vi "Close.vi"(8 "error in (no error)":errorcluster, 11 "Mercury Reference":T1) -> (0 "error out":errorcluster)   [LabVIEW 2019, in "Mercury iXX.lvlib"]
doc: "Close the Mercury reference to the instrument. This will close the physcial communication layer.\nPlease use this only once at the end of your application."
uses:
  Mercury iXX.lvlib
  Controls/Mercury Reference.ctl
  Controls/Comms Transport Layer.ctl
  Private/Controls/Query Dynamic Reference.ctl
  Private/Controls/Lookup Reference FGV Enum.ctl
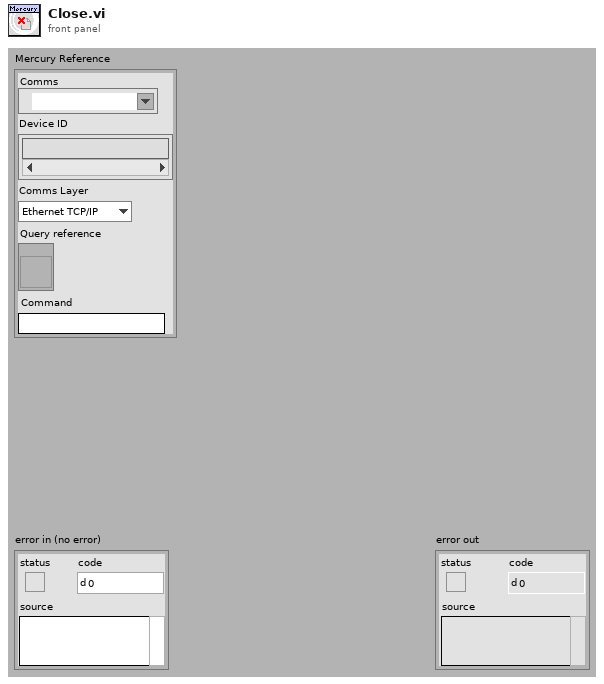
[diagram p1: front panel]
types:
  T1 = typedef "Mercury iXX.lvlib/Mercury Reference.ctl" = cluster{"Comms":refnum<visa-resource-name>, "Device ID":string[], "Comms Layer":T2, "Command":string, "Query reference":T3}
  T2 = typedef "Mercury iXX.lvlib/Comms Transport Layer.ctl" = enum16{"Ethernet TCP/IP", "USB", "ISOBus - RS-232", "GPIB"}
  T3 = typedef "Mercury iXX.lvlib/Query Dynamic Reference.ctl" = refnum<vi>
  T4 = typedef "Mercury iXX.lvlib/Lookup Reference FGV Enum.ctl" = enum16{"Check VISA", "Get VI Ref", "Set VI ref", "Delete Single Ref", "Clear All"}
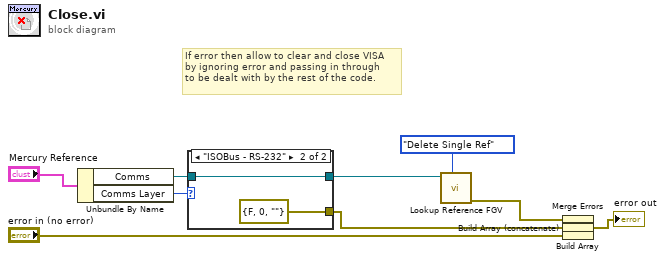
[diagram p0: block diagram]
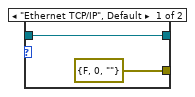
[diagram p2: hidden frame]
diagram:
  # "If error then allow to clear and close VISA\nby ignoring error and passing in through\nto be dealt with by the rest of the code."
  n1 = Unbundle By Name("Mercury Reference") -> ("Comms"=w6:refnum<visa-resource-name>, "Comms Layer"=w8:T2)
  n2 = case shown="\"ISOBus - RS-232\"" w8 {
    tunnel: [errorcluster {"status"=FALSE, "code"=0, "source"=""} ("error out") errorcluster {"status"=FALSE, "code"=0, "source"=""} ("error out")] -> w7
    tunnel: w6 -> [w12 w15]
    tunnel: [w12 w15] -> w4
    frame "Ethernet TCP/IP", Default {
    }
    frame "ISOBus - RS-232" {
    }
  }
  n3 = call "Lookup Reference FGV.vi"("State"=Lookup_Reference_FGV_Enum."Delete Single Ref", "VISA In"=w4) -> ("error out"=w5:errorcluster)  [unwired: 3 in, 6 out]
  n4 = Build Array(w5, w7, "error in (no error)") -> (w2:errorcluster[])
  n5 = Build Array (concatenate)(w2) -> (w1:errorcluster[])
  n6 = Merge Errors(w1) -> (→"error out":errorcluster)
